vi "Simple Reader.vi"(8 "error in (no error)":errorcluster, 11 "SRS Lockin Driver in":refnum<class "SRS Lockin Driver.lvclass">) -> (0 "error out":errorcluster, 2 "Signals":dbl[](array[numeric]), 3 "SRS Lockin Driver out":refnum<class "SRS Lockin Driver.lvclass">)   [LabVIEW 2016, in "SRS Lockin Driver.lvclass"]
uses:
  SRS Lockin Driver.lvclass
  C:/github/NHMFL_Core/Libraries/Instruments/VISA Instrument/VISA Instrument.lvclass
  VISA Instrument/VISA Instrument.lvclass/VISA Instrument.ctl
  VISA Instrument/Read VISA resource.vi
  VISA Instrument/Write VISA resource.vi
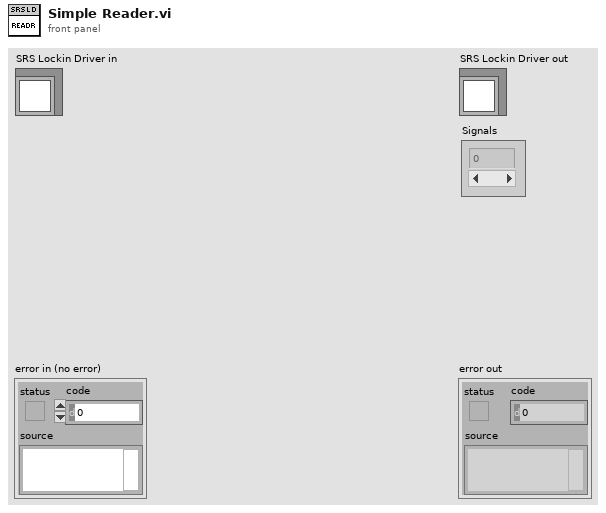
[diagram p1: front panel]
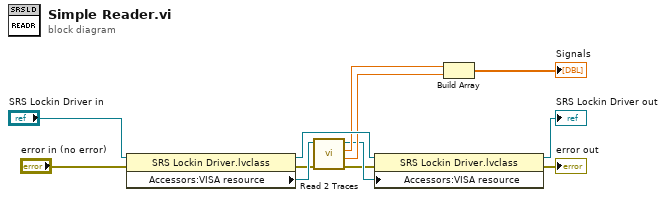
[diagram p0: block diagram]
diagram:
  n1 = property class="SRS Lockin Driver.lvclass"(reference="SRS Lockin Driver in", error in="error in (no error)") -> (reference out=w11:refnum<class "SRS Lockin Driver.lvclass">, error out=w3:errorcluster, "Accessors:VISA resource"=w7:refnum<visa-resource-name>)
  n2 = call "Read 2 Traces.vi"("error in (no error)"=w3, "VISA Resource Name"=w7) -> ("error out"=w2:errorcluster, "Y"=w5:dbl, "X"=w6:dbl, "VISA Resource Name Out"=w4:refnum<visa-resource-name>)  [unwired: 4 in, 2 out]
  n3 = property class="SRS Lockin Driver.lvclass"(reference=w11, error in=w2, "Accessors:VISA resource"=w4) -> (reference out=→"SRS Lockin Driver out":refnum<class "SRS Lockin Driver.lvclass">, error out=→"error out":errorcluster)
  n4 = Build Array(w6, w5) -> (→"Signals":dbl[])
